vi "LabVIEW_Fita_2.2.vi"() -> ()   [LabVIEW 2019]
uses:
  <vilib>/Analysis/5stat.llb/RMS (DBL).vi
  <vilib>/Waveform/WDTOps.llb/WDT Index Channel DBL.vi
  <vilib>/Analysis/NI_AALPro.lvlib
panel:
  in  "Botó d'abortar":bool
  in  "Botó de marxa":bool
  in  "Número de dades per fer mitjana":dbl
  in  "Interval entre dues adquisicions (ms)":dbl
  in  "Durada de l'adquisició (ms)":dbl
  in  "Número de canals a adquirir":dbl
  out "rms value":dbl format="%0.2f"
  out "t0":timestamp
  out "dt":dbl
  out "Valor històric":waveform(dbl)(graph)
  out "Valor actual":dynamicdata(graph)
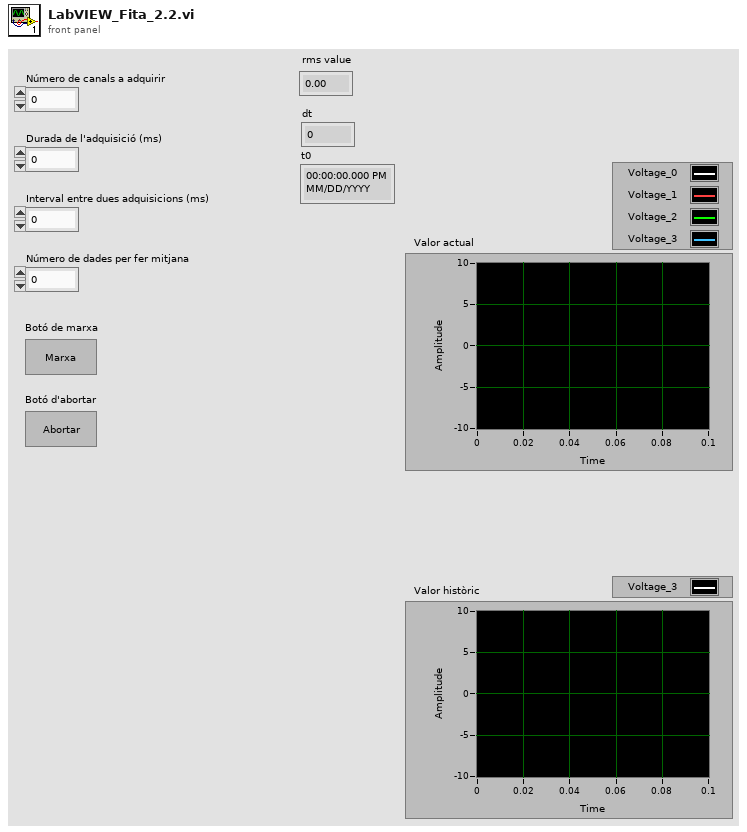
[diagram p1: front panel]
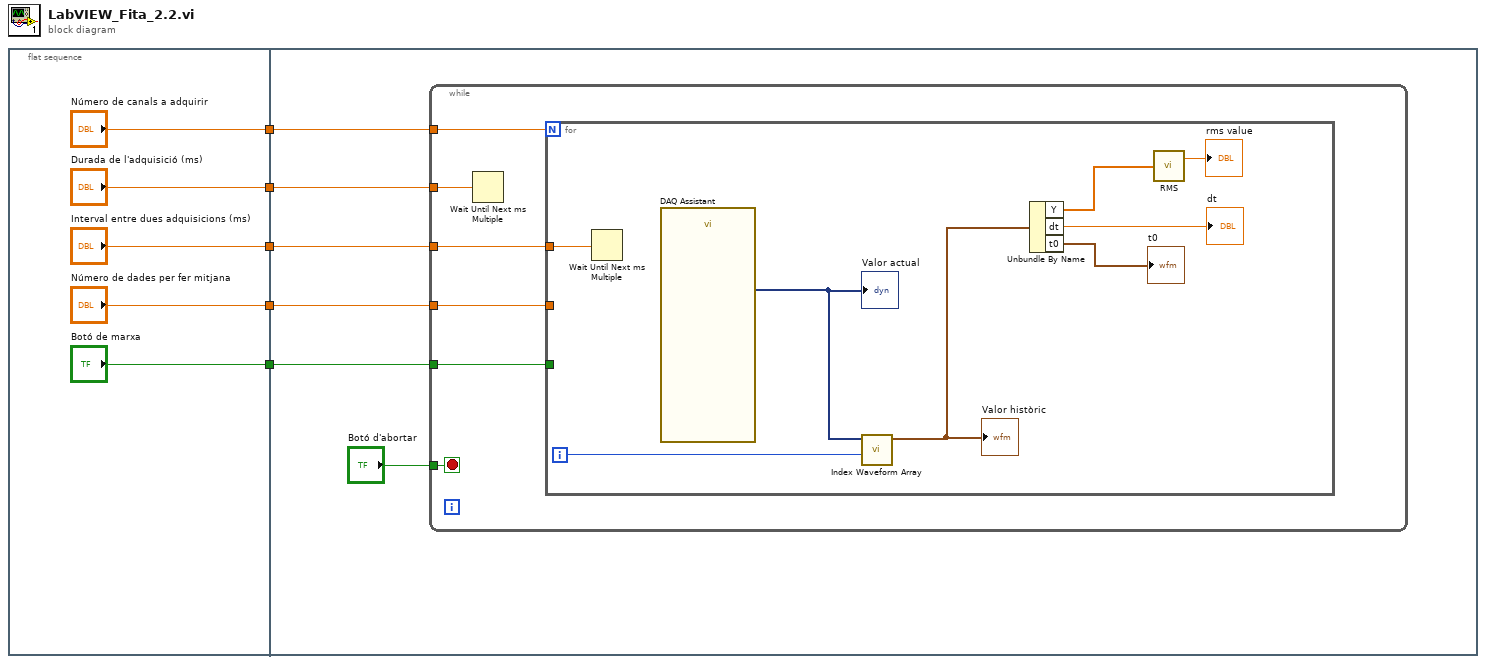
[diagram p0: block diagram]
diagram:
  n1 = flat-sequence {
    tunnel: ["Durada de l'adquisició (ms)"] -> w5
    tunnel: ["Interval entre dues adquisicions (ms)"] -> w4
    tunnel: ["Número de dades per fer mitjana"] -> w3
    tunnel: ["Botó de marxa"] -> w2
    tunnel: ["Número de canals a adquirir"] -> w1
    tunnel: w5 -> [w16]
    tunnel: w4 -> [w15]
    tunnel: w3 -> [w14]
    tunnel: w2 -> [w13]
    tunnel: w1 -> [w12]
    frame #0 {
    }
    frame #1 {
      n2 = while {
        tunnel: w16 -> [w17]
        tunnel: w15 -> [w22]
        tunnel: w14 -> [w21]
        tunnel: w13 -> [w20]
        tunnel: w12 -> [w19]
        tunnel: "Botó d'abortar" -> [w18]
        stop <- w18 stop-if-true
        n3 = Wait Until Next ms Multiple(millisecond multiple=w17) -> ()  [unwired: 1 out]
        n4 = for {
          N: w19 -> [_]
          tunnel: w22 -> [w24]
          tunnel: w21 -> [_]
          tunnel: w20 -> [_]
          i -> [w23]
          n5 = Wait Until Next ms Multiple(millisecond multiple=w24) -> ()  [unwired: 1 out]
          n6 = call "DAQ Assistant"() -> ("data"=w25:dynamicdata)  [unwired: 17 in, 2 out]
          "Valor actual" <- w25
          n7 = call-poly <vilib>:"Index Waveform Array.vi"("index"=w23, "waveform array"=w25) -> ("waveform"=w26:waveform(dbl))  [unwired: 8 in, 1 out]
          "Valor històric" <- w26
          n8 = Unbundle By Name(w26) -> ("Y"=w29:dbl[], "dt"=→"dt":dbl, "t0"=→"t0":timestamp)
          n9 = call-poly <vilib>:"RMS.vi"("X"=w29) -> ("rms value"=→"rms value":dbl)  [unwired: 1 out]
        }
      }
    }
  }
